vi "Global message.vi"() -> ()   [LabVIEW 2021]
panel:
  out "Message":string
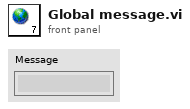
[diagram p1: front panel]
diagram:
